vi "PathPlanner_GoalEndState_Equals.vi"(9 "Other GoalEndState":T1={"Velocity"=0.0, "Rotation"={"VALUE"=0.0, "COS"=1.0, "SIN"=0.0}} {"Rotation"."SIN" format="%13.4f"; "Rotation"."COS" format="%13.4f"; "Rotation"."VALUE" format="%13.4f"}, 11 "GoalEndState":T1={"Velocity"=0.0, "Rotation"={"VALUE"=0.0, "COS"=1.0, "SIN"=0.0}} {"Rotation"."SIN" format="%13.4f"; "Rotation"."COS" format="%13.4f"; "Rotation"."VALUE" format="%13.4f"}) -> (3 "Equal":bool)   [LabVIEW 2019, in "PathPlanner.lvlib"]
doc: "Determines if two Goal End State definitions are equal\n\nInputs:\n -- GoalEndState - cluster - goal end state definition\n -- Other GoalEndState - cluster - goal end state definition\n\nOutputs:\n -- Equal - boolean - TRUE if both definitions are the same."
uses:
  PathPlanner.lvlib
  TypeDef/PathPlannerGoalEndState.ctl
  <vilib>/Rock Robotics/WPI/ThirdParty/JAS_Junk/TrajLib/TypeDef/ROTATION2D.ctl
  <vilib>/Rock Robotics/WPI/ThirdParty/JAS_Junk/TrajLib/Util_CalcDist.vi
  <vilib>/Rock Robotics/WPI/ThirdParty/JAS_Junk/TrajLib/Trajectory_Library.lvlib
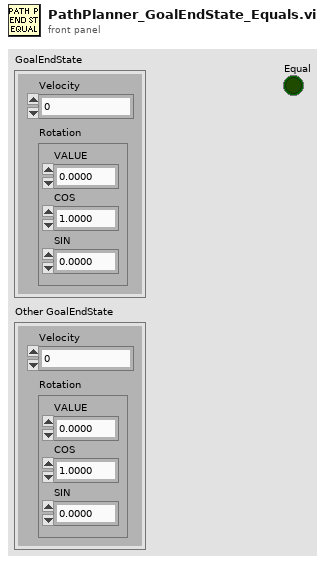
[diagram p1: front panel]
types:
  T1 = typedef "PathPlanner.lvlib/PathPlannerGoalEndState.ctl" = cluster{"Velocity":dbl, "Rotation":T2}
  T2 = typedef "Trajectory_Library.lvlib/ROTATION2D.ctl" = cluster{"VALUE":dbl, "COS":dbl, "SIN":dbl}
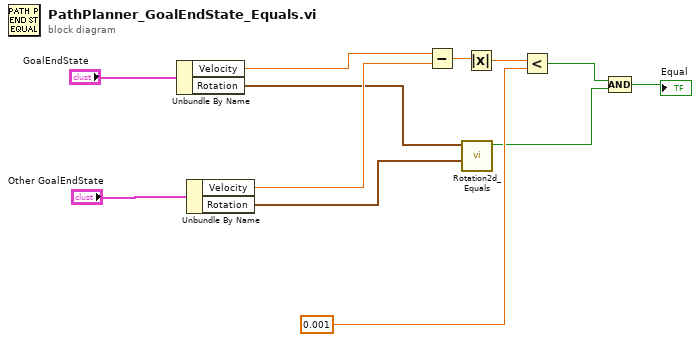
[diagram p0: block diagram]
diagram:
  n1 = Unbundle By Name("GoalEndState") -> ("Velocity"=w10:dbl, "Rotation"=w3:T2)
  n2 = Unbundle By Name("Other GoalEndState") -> ("Velocity"=w9:dbl, "Rotation"=w2:T2)
  n3 = Subtract(x=w10, y=w9) -> (x-y=w8:dbl)
  n4 = call <vilib>:"Rotation2d_Equals.vi"("other ROTATION"=w2, "in ROTATION"=w3) -> ("Equals"=w1:bool)  [unwired: 9 in]
  n5 = Absolute Value(x=w8) -> (abs(x)=w7:dbl)
  n6 = Less?(x=w7, y=0.001) -> (x < y?=w6:bool)
  n7 = Compound Arithmetic op=AND(w6, w1) -> (→"Equal":bool)
